vi "Project.vi"() -> ()   [LabVIEW 2020]
uses:
  <vilib>/Analysis/3filter.llb/Filter Passband Type.ctl
  <vilib>/Instr/_visa.llb/VISA Configure Serial Port (Instr).vi
  <vilib>/ptbypt/NI_PtbyPt.lvlib
  <vilib>/Analysis/NI_AALBase.lvlib
panel:
  out "Left Arm Binary":dbl(graph)
  in  "Virtual Key":u8(ring)=65
  out "Right Arm Binary":dbl(graph)
  in  "VISA resource name":refnum<visa-resource-name>
  in  "baud rate":u32=9600
  out "Available?":bool
  in  "Knob":i64(knob) scale=0.0..2.0
  out "String":string
  out "Concactenate String":string
  out "Index Number":u32
  out "Button Pressed":u8(graph)
  out "Serial Settings:Number of Bytes at Serial Port":u32
  in  "stop":bool
  out "Index":i32
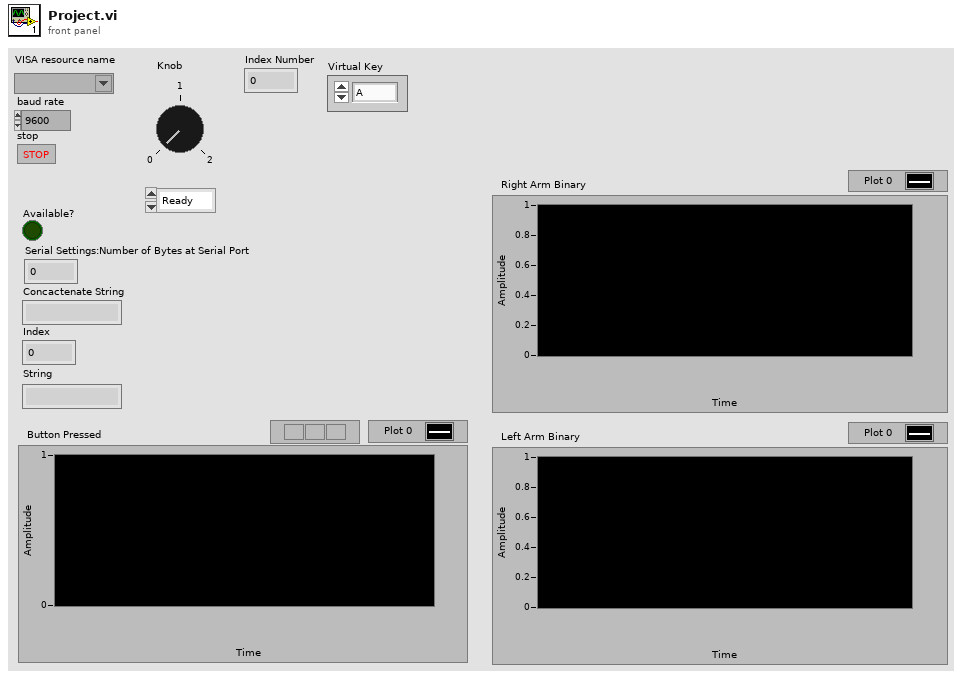
[diagram p1: front panel]
types:
  T1 = typedef "NI_AALBase.lvlib/Filter Passband Type.ctl" = enum32{"Lowpass", "Highpass", "Bandpass", "Bandstop"}
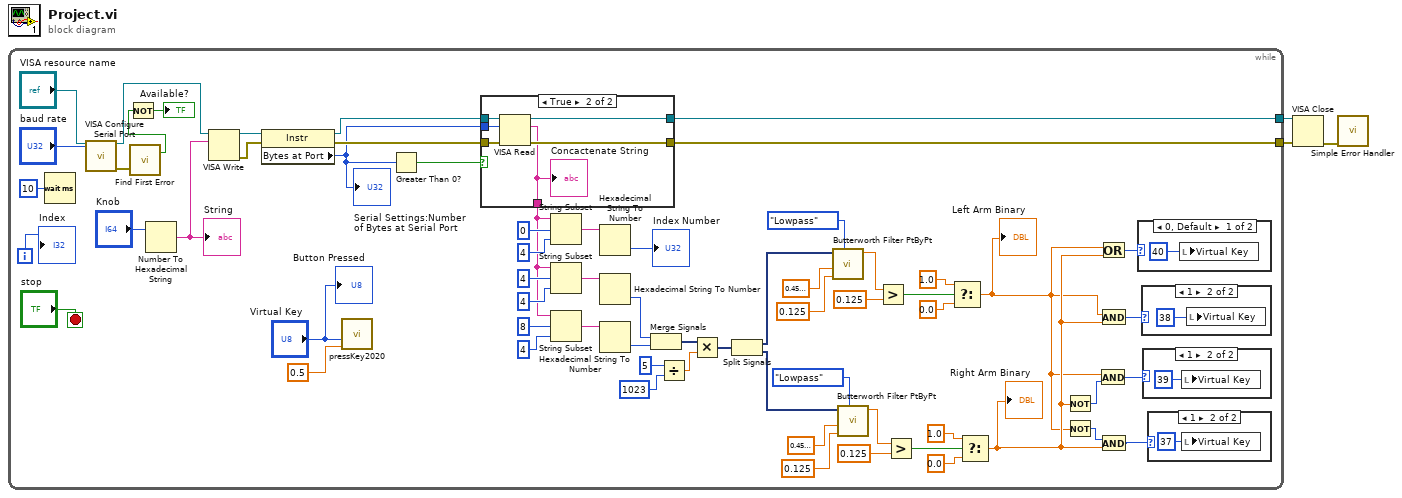
[diagram p0: block diagram]
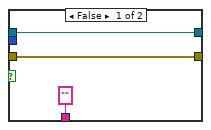
[diagram p6: hidden frame]
diagram:
  n1 = while {
    tunnel: [w54] -> w3
    tunnel: [w53] -> w2
    i -> [w56]
    stop <- "stop" stop-if-true
    n2 = Wait (ms)(milliseconds to wait=10) -> ()  [unwired: 1 out]
    n3 = call-poly "VISA Configure Serial Port"("VISA resource name"="VISA resource name", "baud rate (9600)"="baud rate") -> ("VISA resource name out"=w64:refnum<visa-resource-name>, "error out"=w66:errorcluster)  [unwired: 12 in]
    n4 = call <vilib>:"Find First Error.vi"("error in (no error)"=w66) -> ("error?"=w51:bool)  [unwired: 3 in, 1 out]
    n5 = Not(x=w51) -> (.not. x?=→"Available?":bool)
    n6 = Number To Hexadecimal String(2:"Knob") -> (0:w62:string)  [unwired: 1 in]
    "String" <- w62
    n7 = VISA Write(VISA resource name=w64, write buffer=w62) -> (VISA resource name out=w61:refnum<visa-resource-name>, error out=w60:errorcluster)  [unwired: 1 in, 1 out]
    n8 = property class="Instr"(reference=w61, error in=w60) -> (reference out=w59:refnum<visa-resource-name>, error out=w55:errorcluster, "Bytes at Port"=w50:u32)
    "Serial Settings:Number of Bytes at Serial Port" <- w50
    n9 = call "pressKey2020.vi"("time"=0.5, "Virtual Key"="Virtual Key") -> ()  [unwired: 10 in]
    n10 = Greater Than 0?(x=w50) -> (x > 0?=w58:bool)
    n11 = case shown="True" w58 {
      tunnel: w59 -> [w75 w81]
      tunnel: w50 -> [_ w80]
      tunnel: [w75 w79] -> w54
      tunnel: [w74 w78] -> w53
      tunnel: w55 -> [w74 w77]
      tunnel: ["" ("read buffer") w76] -> w39
      frame False {
      }
      frame True {
        n12 = VISA Read(VISA resource name=w81, byte count=w80, error in (no error)=w77) -> (VISA resource name out=w79:refnum<visa-resource-name>, read buffer=w76:string, error out=w78:errorcluster)  [unwired: 1 out]
        "Concactenate String" <- w76
      }
    }
    n13 = String Subset(string=w39, offset (0)=0, length (rest)=4) -> (substring=w47:string)
    n14 = String Subset(string=w39, offset (0)=4, length (rest)=4) -> (substring=w48:string)
    n15 = String Subset(string=w39, offset (0)=8, length (rest)=4) -> (substring=w40:string)
    n16 = Hexadecimal String To Number(string=w47) -> (number=→"Index Number":u32)  [unwired: 2 in, 1 out]
    n17 = Hexadecimal String To Number(string=w48) -> (number=w27:u32)  [unwired: 2 in, 1 out]
    n18 = Hexadecimal String To Number(string=w40) -> (number=w26:u32)  [unwired: 2 in, 1 out]
    n19 = Merge Signals(w27, w26) -> (w25:dynamicdata)
    n20 = Divide(x=5, y=1023) -> (x/y=w36:dbl)
    n21 = Multiply(x=w25, y=w36) -> (x*y=w13:dynamicdata)
    n22 = Split Signals(w13) -> (w21:dynamicdata, w20:dynamicdata)  [unwired: 2 in]
    n23 = call <vilib>:"Butterworth Filter PtByPt.vi"("filter type"=Filter_Passband_Type."Lowpass", "low cutoff freq: fl"=0.125, "high cutoff freq: fh"=0.45000000000000007, "x"=w21) -> ("Filtered x"=w16:dbl)  [unwired: 5 in, 1 out]
    n24 = call <vilib>:"Butterworth Filter PtByPt.vi"("filter type"=Filter_Passband_Type."Lowpass", "low cutoff freq: fl"=0.125, "high cutoff freq: fh"=0.45000000000000007, "x"=w20) -> ("Filtered x"=w28:dbl)  [unwired: 5 in, 1 out]
    n25 = Greater?(x=w16, y=0.125) -> (0:w18:bool)
    n26 = Greater?(x=w28, y=0.125) -> (0:w31:bool)
    n27 = Select(t=1.0, s=w18, f=0.0) -> (s? t:f=w5:dbl)
    "Left Arm Binary" <- w5
    n28 = Select(t=1.0, s=w31, f=0.0) -> (s? t:f=w9:dbl)
    "Right Arm Binary" <- w9
    n29 = Not(x=w9) -> (.not. x?=w10:u32)
    n30 = Not(x=w5) -> (.not. x?=w11:u32)
    n31 = And(x=w5, y=w10) -> (x .and. y?=w7:i32)
    n32 = Or(x=w5, y=w9) -> (x .or. y?=w6:i32)
    n33 = And(x=w5, y=w9) -> (x .and. y?=w8:i32)
    n34 = And(x=w11, y=w9) -> (x .and. y?=w12:i32)
    n35 = case shown="0, Default" w6 {
      frame 0, Default {
        n36 = local write "Virtual Key"(40) -> ()
      }
      frame 1 {
      }
    }
    n37 = case shown="1" w8 {
      frame 0, Default {
      }
      frame 1 {
        n38 = local write "Virtual Key"(38) -> ()
      }
    }
    n39 = case shown="1" w7 {
      frame 0, Default {
      }
      frame 1 {
        n40 = local write "Virtual Key"(39) -> ()
      }
    }
    n41 = case shown="1" w12 {
      frame 0, Default {
      }
      frame 1 {
        n42 = local write "Virtual Key"(37) -> ()
      }
    }
    "Index" <- w56
    "Button Pressed" <- "Virtual Key"
  }
  n43 = VISA Close(VISA resource name=w3, error in (no error)=w2) -> (error out=w1:errorcluster)
  n44 = call <vilib>:"Simple Error Handler.vi"("error in (no error)"=w1) -> ()  [unwired: 4 in, 5 out]
